vi "driveShifter.vi"(10 "?":T1) -> ()   [LabVIEW 2018]
uses:
  driveShifterEnum.ctl
  <vilib>/Rock Robotics/WPI/Solenoid/WPI_SolenoidValue.ctl
  <userlib>/836-Library/System/TDMS_V2/Support/TDMS_DevRef.ctl
  <userlib>/836-Library/System/TDMS_V2/Support/Logging_Settings.ctl
  <userlib>/836-Library/System/TDMS_V2/Support/Group_FIFO_Config.ctl
  <userlib>/836-Library/System/TDMS_V2/Support/Channel_FIFO_Config.ctl
  <vilib>/Rock Robotics/WPI/Solenoid/WPI_SolenoidSetEnum.vi
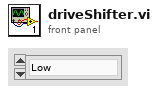
[diagram p1: front panel]
types:
  T1 = typedef "driveShifterEnum.ctl" = enum16{"Low", "High"}
  T2 = typedef "TDMS_DevRef.ctl" = cluster{"Name":string, "File Ref":refnum<k34>, "Start Time":timestamp, "Logging Settings":T3, "Group FIFO Config":T4[], "Data To Write":refnum<data-value>, "semaphore":T6, "Ref Time Reset":refnum<k4>}
  T3 = typedef "Logging_Settings.ctl" = cluster{"Data Grab Period":dbl, "File Write Period":dbl, "Max Stored Size":dbl, "Burst Size":dbl}
  T4 = typedef "Group_FIFO_Config.ctl" = cluster{"Group":string, "Channels":T5[], "Channel Names":string[]}
  T5 = typedef "Channel_FIFO_Config.ctl" = cluster{"Channel":string, "FIFO":refnum<k33>}
  T6 = typedef "Semaphore RefNum" = refnum<k1>
  T7 = typedef "WPI_SolenoidValue.ctl" = enum16{"Off", "On", "Forward", "Reverse"}
  T8 = typedef "WPI_SolenoidDevRef.ctl" = cluster{"DevStatus":errorcluster, "Pneumatics Control Module":u8, "Forward Solenoid Channel":T9, "Reverse Solenoid Channel":T9}
  T9 = typedef "WPI_SolenoidChannel.ctl" = enum8{"Solenoid 0", "Solenoid 1", "Solenoid 2", "Solenoid 3", "Solenoid 4", "Solenoid 5", "Solenoid 6", "Solenoid 7", "Invalid"}
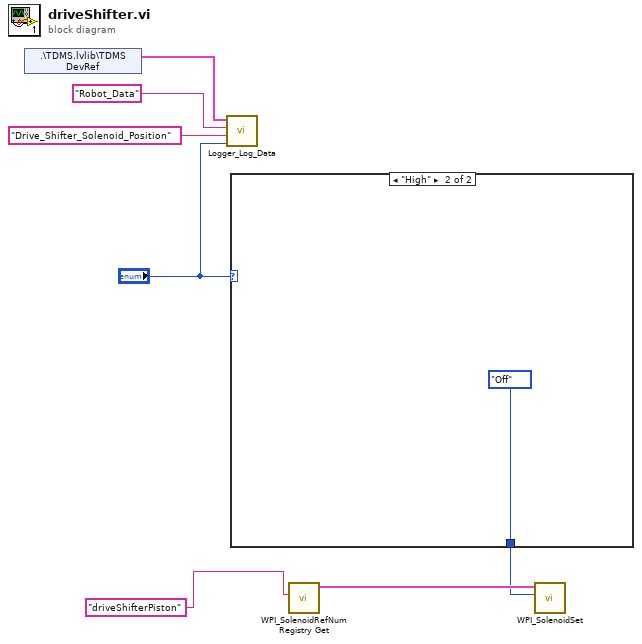
[diagram p0: block diagram]
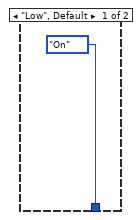
[diagram p2: hidden frame]
diagram:
  n1 = shared-variable ".\\TDMS.lvlib\\TDMS DevRef"() -> (w2:T2)  [unwired: 1 in, 1 out]
  n2 = call <userlib>:"Logger_Log_Data.vi"("Data"="?", "Channel"="Drive_Shifter_Solenoid_Position", "Group"="Robot_Data", "TDMS DevRef"=w2) -> ()  [unwired: 7 in, 1 out]
  n3 = case shown="\"High\"" "?" {
    tunnel: [WPI_SolenoidValue."On" ("Value") WPI_SolenoidValue."Off" ("Value")] -> w6
    frame "Low", Default {
    }
    frame "High" {
    }
  }
  n4 = call <vilib>:"WPI_SolenoidRefNum Registry Get.vi"("refnum name"="driveShifterPiston") -> ("SolenoidDevRef"=w7:T8)  [unwired: 9 in, 1 out]
  n5 = call-poly <vilib>:"WPI_SolenoidSet.vi"("Value"=w6, "SolenoidDevRef"=w7) -> ()  [unwired: 8 in, 2 out]
